vi "ble_read_write_characteristics.vi"() -> ()   [LabVIEW 2015]
uses:
  <vilib>/BLE/type_def/connection_status_bundle.ctl
  <vilib>/BLE/type_def/address_type.ctl
  <vilib>/BLE/ble_functions/ble_write_by_service_characteristic_uint8array.vi
  <vilib>/BLE/ble_functions/ble_write_by_handle_uint8array.vi
panel:
  out "숫자형":i32
  in  "Rx 정지":bool
  out "Rx 문자열":string
  out "Connected":bool
  out "Device Name":string
  in  "Address Type":T1 items=["Public", "Random"]
  out "Handle table":string[][](array[string])
  out "Connection Status":T2={"MAC Address"="00:17:EA:91:6D:C6", "cnx handle"=0, "cnx flags"=5, "Address Type"=0, "Connection Interval (ms)"=75, "Timeout(ms)"=1000, "Latency"=0, "bonding handle"=255} {"Address Type" items=["Public", "Random"]}
  out "Scanning":bool
  in  "Continue":bool
  in  "MAC Address":string="00:17:EA:91:6D:C6"
  in  "COM Bluegiga in":refnum<visa-resource-name>="COM8"
  out "Devices":string[][](array[string])
  out "BLED112 Dongle Info":string
  # "connection_status_bundle.ctlThis VI an example of scanning for BLE devices using the \nBLED112 Bluetooth Smart Dongle by Bluegiga\nhttps://www.bluegiga.com/en-US/products/bled112-bluetooth-smart-dongle/\n\nand\nBLE (Bluetooth Low Energy) toolkit for LabVIEW\nww.\n\nInstructions:\nBefore running the VI\n1. Select the COM port for the BLED112 USB receiver\n(You can verify this in the Device Manager)\n\n2. Run the VI\n\n3. The VI will reset the dongle and scan for available BLE devices\n \n4. Introduce the MAC Address and Address Type of the device you want to connect and click in the CONTINUE button to connect with it\n\n5. The VI will read the Characteristic 0x2A00 of the Service 0x1800 which contains \nthe Device Name\n\nhttps://www.bluetooth.com/specifications/gatt/viewer?attributeXmlFile=org.bluetooth.service.generic_access.xml&u=org.bluetooth.service.generic_access.xml"
  # "SCAN"
  # "RSSI (power)"
  # "Advertising Package Type"
  # "MAC Address"
  # "Address Type"
  # "Friendly name"
  # "DEVICES FOUND"
  # "Introduce the MAC Address and Address Type of the device you want to connect and click in the CONTINUE button"
  # "CONNECT"
  # "READING DEVICE NAME"
  # "Service 0x1800\nCharacteristic 0x2A00\nDevice Name"
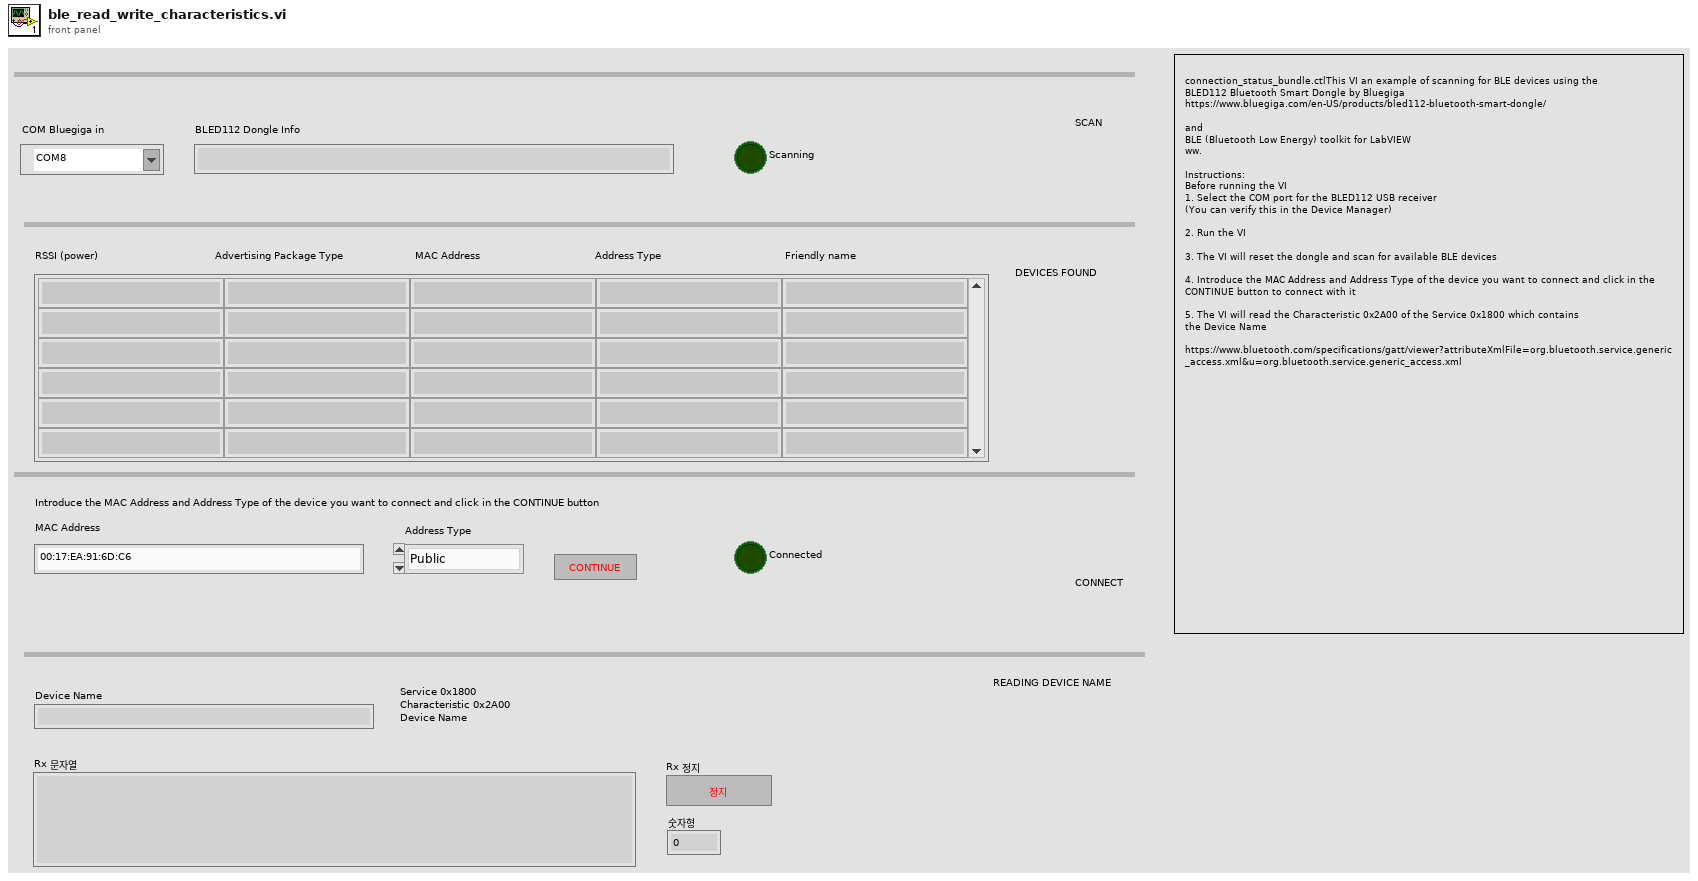
[diagram p1: front panel]
types:
  T1 = typedef "address_type.ctl" = u8
  T2 = typedef "connection_status_bundle.ctl" = cluster{"MAC Address":string, "cnx handle":u8, "cnx flags":u8, "Address Type":T1, "Connection Interval (ms)":u16, "Timeout(ms)":u16, "Latency":u16, "bonding handle":u8}
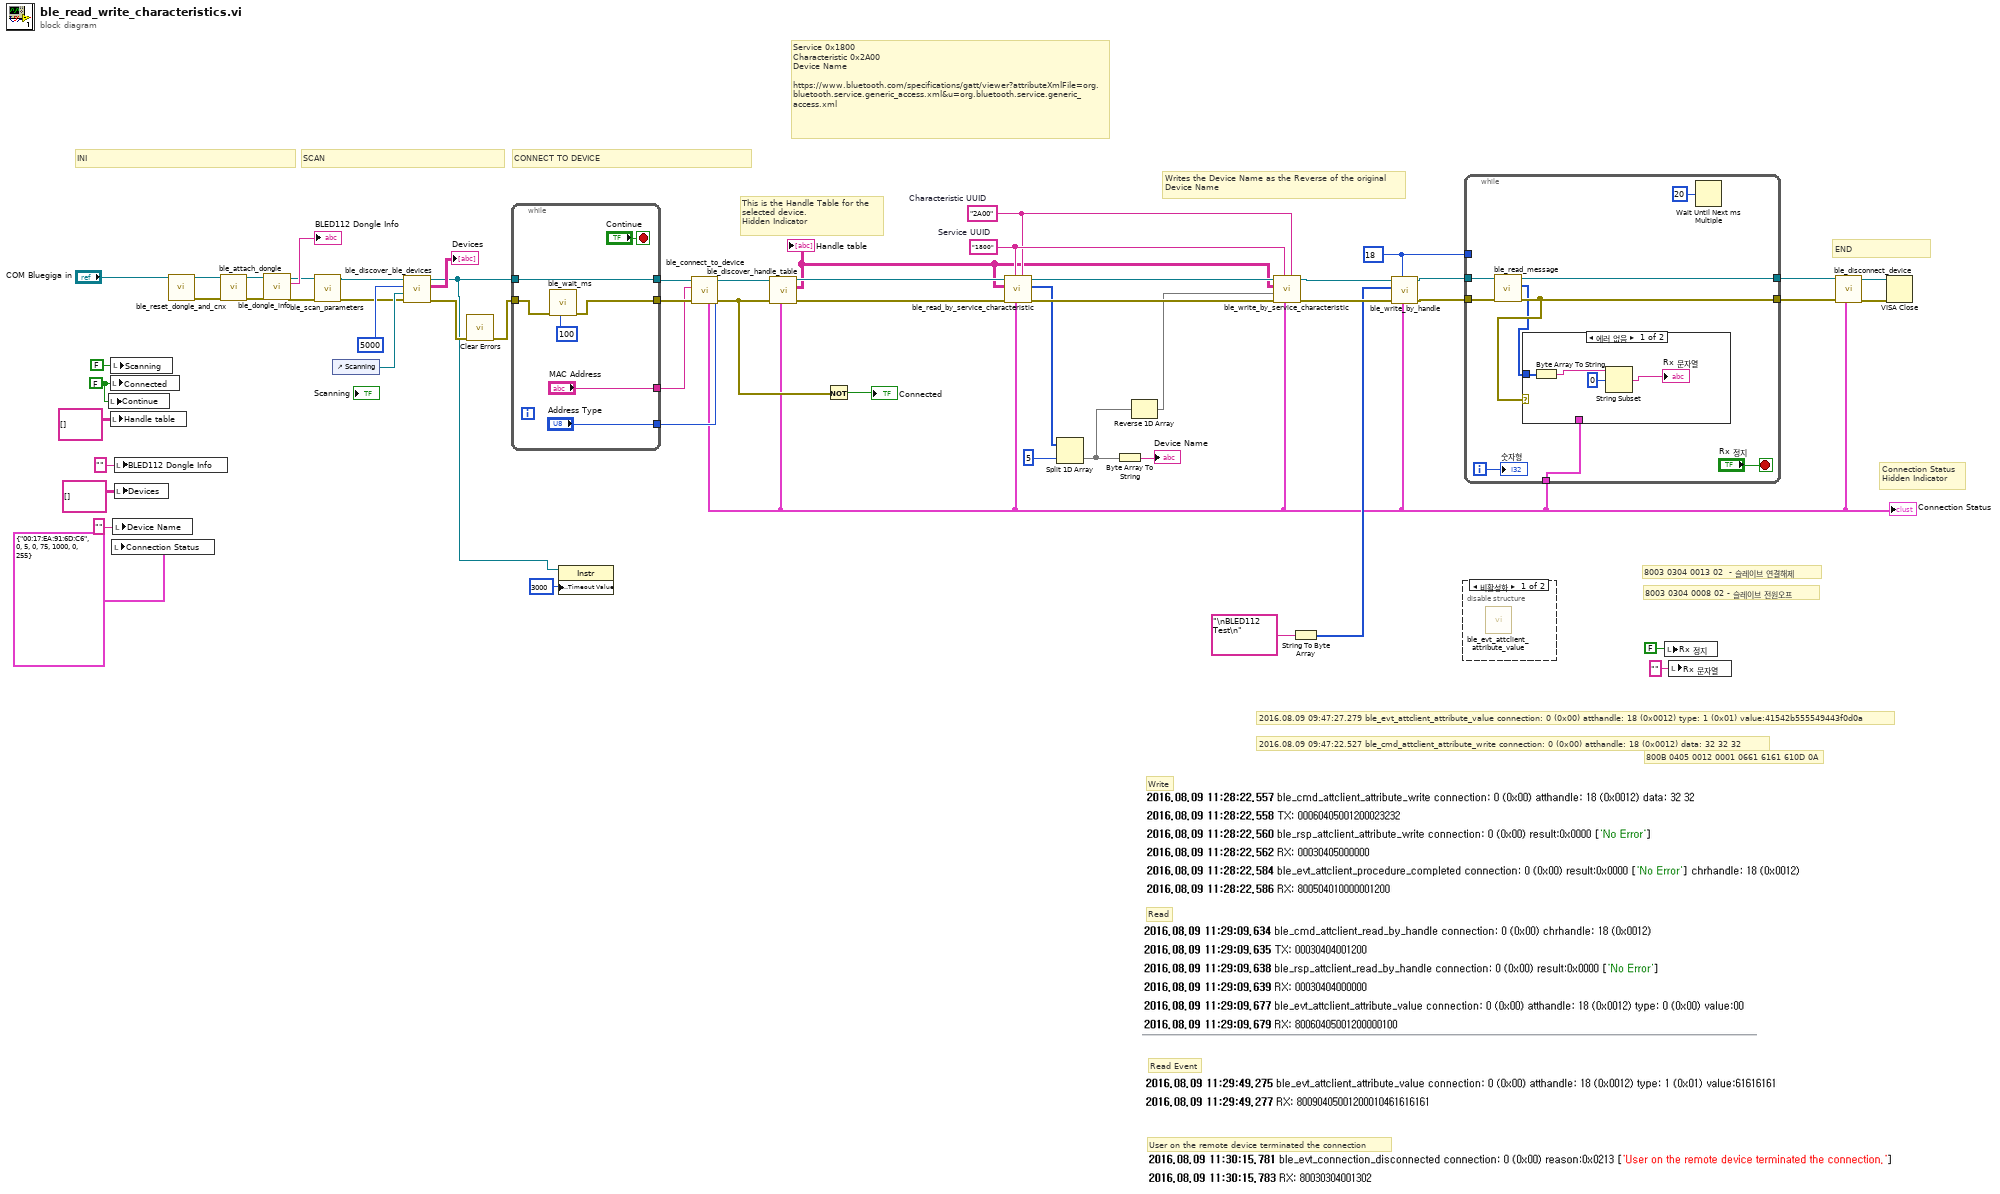
[diagram p0: block diagram]
diagram:
  w10 = u16 18 ("Handle")
  w21 = FALSE ("Connected")
  w27 = "2A00"  # Characteristic UUID
  w28 = "1800"  # Service UUID
  # "8003 0304 0008 02 - 슬레이브 전원오프"
  # "8003 0304 0013 02  - 슬레이브 연결해제"
  # "User on the remote device terminated the connection"
  # "Read Event"
  # "Read"
  # "Write"
  # "800B 0405 0012 0001 0661 6161 610D 0A"
  # "2016.08.09 09:47:22.527 ble_cmd_attclient_attribute_write connection: 0 (0x00) atthandle: 18 (0x0012) data: 32 32 32"
  # "2016.08.09 09:47:27.279 ble_evt_attclient_attribute_value connection: 0 (0x00) atthandle: 18 (0x0012) type: 1 (0x01) value:41542b555549443f0d0a"
  # "Writes the Device Name as the Reverse of the original\nDevice Name"
  # "Connection Status\nHidden Indicator"
  # "Service 0x1800\nCharacteristic 0x2A00\nDevice Name\n\nhttps://www.bluetooth.com/specifications/gatt/viewer?attributeXmlFile=org.bluetooth.service.generic_access.xml&u=org.bluetooth.service.generic_access.xml"
  # "This is the Handle Table for the\nselected device. \nHidden Indicator"
  # "CONNECT TO DEVICE"
  # "SCAN"
  # "END"
  # "INI"
  n1 = local write "Continue"(w21) -> ()
  n2 = local write "Connected"(w21) -> ()
  n3 = local write "Handle table"(string[][] [] ("Handle table")) -> ()
  n4 = local write "Scanning"(FALSE ("Scanning")) -> ()
  n5 = local write "Connection Status"(T2 {"MAC Address"="00:17:EA:91:6D:C6", "cnx handle"=0, "cnx flags"=5, "Address Type"=0, "Connection Interval (ms)"=75, "Timeout(ms)"=1000, "Latency"=0, "bonding handle"=255} ("Connection Status")) -> ()
  n6 = local write "Device Name"("" ("Device Name")) -> ()
  n7 = local write "BLED112 Dongle Info"("" ("BLED112 Dongle Info")) -> ()
  n8 = local write "Devices"(string[][] [] ("Devices")) -> ()
  n9 = call <vilib>:"ble_reset_dongle_and_cnx.vi"("COM Bluegiga in"="COM Bluegiga in") -> ("error out"=w42:errorcluster, "COM Bluegiga out"=w41:refnum<visa-resource-name>)  [unwired: 9 in]
  n10 = call <vilib>:"ble_attach_dongle.vi"("error in (no error)"=w42, "COM Bluegiga in"=w41) -> ("error out"=w44:errorcluster, "COM Bluegiga out"=w43:refnum<visa-resource-name>)  [unwired: 8 in]
  n11 = call <vilib>:"ble_dongle_info.vi"("error in (no error)"=w44, "COM Bluegiga in"=w43) -> ("error out"=w50:errorcluster, "info"=→"BLED112 Dongle Info":string, "COM Bluegiga out"=w51:refnum<visa-resource-name>)  [unwired: 7 in]
  n12 = call <vilib>:"ble_scan_parameters.vi"("error in (no error)"=w50, "COM Bluegiga in"=w51) -> ("error out"=w48:errorcluster, "COM Bluegiga out"=w49:refnum<visa-resource-name>)  [unwired: 7 in, 1 out]
  n13 = control-ref of="Scanning"() -> (w54:refnum<vi>)
  n14 = call <vilib>:"ble_discover_ble_devices.vi"("error in (no error)"=w48, "LED ref"=w54, "Scan Duration (10000ms)"=u32 5000, "COM Bluegiga in"=w49) -> ("error out"=w39:errorcluster, "Devices"=→"Devices":string[][], "COM Bluegiga out"=w1:refnum<visa-resource-name>)  [unwired: 5 in]
  n15 = call <vilib>:"Clear Errors.vi"("error in (no error)"=w39) -> ("error out"=w38:errorcluster)  [unwired: 5 in, 1 out]
  n16 = while {
    tunnel: w38 -> [w63]
    tunnel: [w62] -> w53
    tunnel: w1 -> [w62]
    tunnel: [w61] -> w52
    tunnel: ["MAC Address"] -> w45
    tunnel: ["Address Type"] -> w37
    stop <- "Continue" stop-if-true
    n17 = call <vilib>:"ble_wait_ms.vi"("milliseconds to wait (100)"=u32 100, "error in (no error)"=w63) -> ("error out"=w61:errorcluster)  [unwired: 9 in]
  }
  n18 = property class="Instr"(reference=w1, "General Settings:Timeout Value"=u32 3000) -> ()  [unwired: 1 in, 2 out]
  n19 = call <vilib>:"ble_connect_to_device.vi"("Address Type"=w37, "error in (no error)"=w52, "MAC Address"=w45, "COM Bluegiga in"=w53) -> ("error out"=w31:errorcluster, "COM Bluegiga out"=w40:refnum<visa-resource-name>, "Connection Status"=w12:T2)  [unwired: 5 in]
  "Connection Status" <- w12
  n20 = call <vilib>:"ble_discover_handle_table.vi"("Connection Status"=w12, "error in (no error)"=w31, "COM Bluegiga in"=w40) -> ("error out"=w36:errorcluster, "Handle table"=w26:string[][], "COM Bluegiga out"=w35:refnum<visa-resource-name>)  [unwired: 6 in]
  "Handle table" <- w26
  n21 = Not(x=w31) -> (.not. x?=→"Connected":bool)
  n22 = call <vilib>:"ble_read_by_service_characteristic.vi"("Characteristic UUID"=w27, "Connection Status"=w12, "Service UUID"=w28, "error in (no error)"=w36, "Handle table"=w26, "COM Bluegiga in"=w35) -> ("error out"=w29:errorcluster, "characteristic value"=w25:u8[], "COM Bluegiga out"=w30:refnum<visa-resource-name>)  [unwired: 3 in]
  n23 = Split 1D Array(array=w25, index=5) -> (second subarray=w24:u8[])  [unwired: 1 out]
  n24 = Byte Array To String(unsigned byte array=w24) -> (string=→"Device Name":string)
  n25 = Reverse 1D Array(array=w24) -> (reversed array=w23:u8[])
  n26 = call-poly <vilib>:"ble_write_by_service_characteristic.vi"("Characteristic UUID"=w27, "Connection Status"=w12, "Service UUID"=w28, "error in (no error)"=w29, "data"=w23, "Handle table"=w26, "COM Bluegiga in"=w30) -> ("error out"=w15:errorcluster, "COM Bluegiga out"=w16:refnum<visa-resource-name>)  [unwired: 3 in]
  n27 = String To Byte Array(string="\nBLED112 Test\n") -> (unsigned byte array=w13:u8[])
  n28 = call-poly <vilib>:"ble_write_by_handle.vi"("Connection Status"=w12, "Handle"=w10, "error in (no error)"=w15, "data (uint8array)"=w13, "COM Bluegiga in"=w16) -> ("error out"=w8:errorcluster, "COM Bluegiga out"=w4:refnum<visa-resource-name>)  [unwired: 5 in]
  n29 = disable-structure shown="비활성화" {
    frame Disabled {
      n30 = call <vilib>:"ble_evt_attclient_attribute_value.vi"() -> ()  [unwired: 8 in, 4 out]
    }
    frame Enabled {
    }
  }
  n31 = while {
    tunnel: w12 -> [w71]
    tunnel: w10 -> [_]
    tunnel: w4 -> [w68]
    tunnel: w8 -> [w69]
    tunnel: [w67] -> w7
    tunnel: [w66] -> w6
    i -> [w70]
    stop <- "Rx 정지" stop-if-true
    n32 = call <vilib>:"ble_read_message.vi"("error in (no error)"=w69, "COM Bluegiga in"=w68) -> ("error out"=w66:errorcluster, "message package"=w65:u8[], "COM Bluegiga out"=w67:refnum<visa-resource-name>)  [unwired: 7 in]
    n33 = case shown="에러 없음" w66 {
      tunnel: w71 -> [_ _]
      tunnel: w65 -> [w77 _]
      frame No Error {
        n34 = Byte Array To String(unsigned byte array=w77) -> (string=w76:string)
        n35 = String Subset(string=w76, offset (0)=0 ("오프셋(0)")) -> (substring=→"Rx 문자열":string)  [unwired: 1 in]
      }
      frame Error {
      }
    }
    n36 = Wait Until Next ms Multiple(millisecond multiple=u32 20 ("ms 배수")) -> ()  [unwired: 1 out]
    "숫자형" <- w70
  }
  n37 = local write "Rx 정지"(FALSE ("Rx 정지")) -> ()
  n38 = local write "Rx 문자열"("" ("Rx 문자열")) -> ()
  n39 = call <vilib>:"ble_disconnect_device.vi"("Connection Status"=w12, "error in (no error)"=w6, "COM Bluegiga in"=w7) -> ("error out"=w46:errorcluster, "COM Bluegiga out"=w47:refnum<visa-resource-name>)  [unwired: 7 in]
  n40 = VISA Close(VISA resource name=w47, error in (no error)=w46) -> ()  [unwired: 1 out]
